vi "ModuleAction.Utility.vi"() -> ()   [LabVIEW 2014]
uses:
  <userlib>/_OpenG.lib/file/file.llb/Strip Path - Traditional__ogtk.vi
panel:
  in  "Stop Button":bool
  in  "Disk Properties":T1
  in  "Action Descriptor":T2
  out "Preview":string
  in  "Write to Disk":bool
  in  "Refresh":bool caption="Blank Button"
  out "Constructed Module Action Descriptor Location:":string
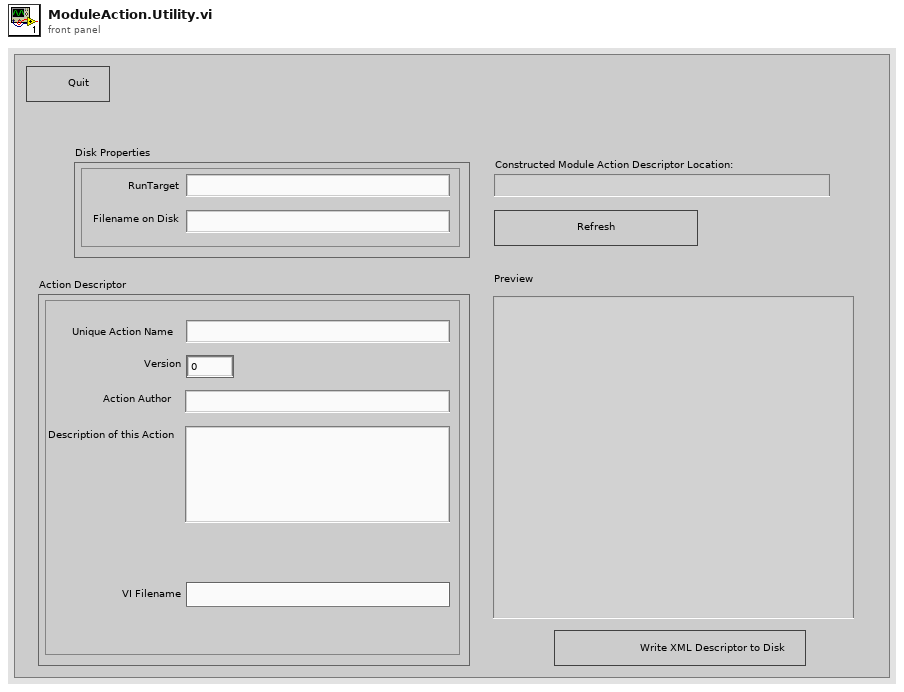
[diagram p1: front panel]
types:
  T1 = cluster{"RunTarget":string, "Filename on Disk":string}
  T2 = cluster{"Unique Action Name":string, "Version":dbl, "VI Filename":string, "Action Author":string, "Description of this Action":string}
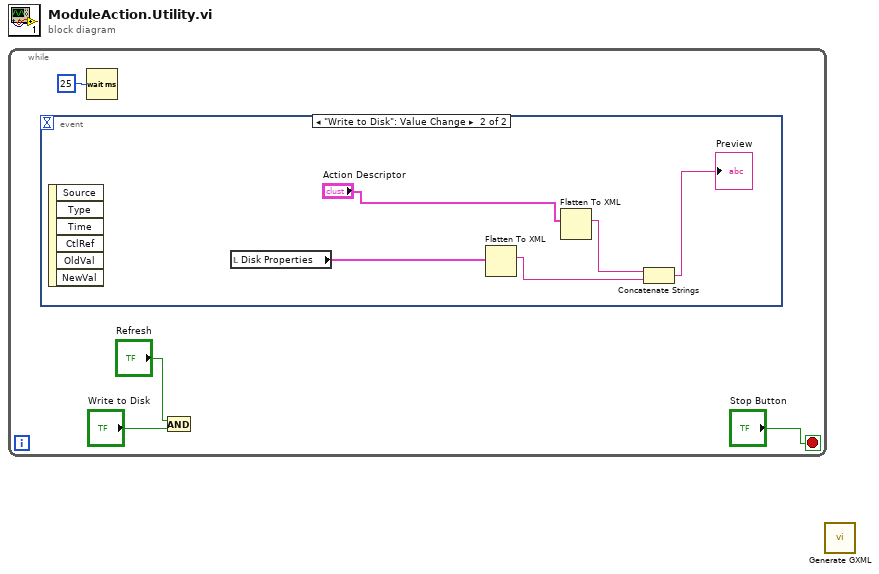
[diagram p0: block diagram]
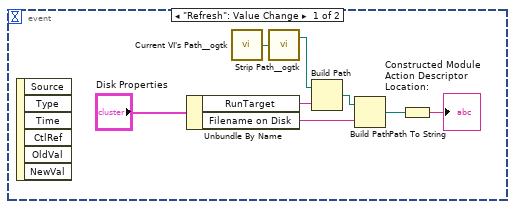
[diagram p2: hidden frame]
diagram:
  n1 = while {
    stop <- "Stop Button" stop-if-true
    n2 = event shown="[1] \"Write to Disk\": Value Change" {
      selector: _ -> [_ _]
      dyn-events: _ -> [_ _]
      timeout: _ -> [_ _]
      event "Refresh": Value Change {
        n3 = event-data() -> ()  [unwired: 1 in, 6 out]
        n4 = Unbundle By Name("Disk Properties") -> ("RunTarget"=w9:string, "Filename on Disk"=w7:string)
        n5 = call <userlib>:"Current VI's Path__ogtk.vi"() -> ("Current VI's Path (+ Relative)"=w11:path)  [unwired: 1 in]
        n6 = call-poly <userlib>:"Strip Path__ogtk.vi"("path"=w11) -> ("stripped path"=w10:path)  [unwired: 1 out]
        n7 = Build Path(base path=w10, name or relative path=w9) -> (appended path=w8:path)
        n8 = Build Path(base path=w8, name or relative path=w7) -> (appended path=w6:path)
        n9 = Path To String(path=w6) -> (string=→"Constructed Module Action Descriptor Location:":string)
      }
      event "Write to Disk": Value Change {
        n10 = event-data() -> ()  [unwired: 1 in, 6 out]
        n11 = local read "Disk Properties"() -> (w14:T1)
        n12 = Flatten To XML(anything=w14) -> (xml string=w13:string)
        n13 = Flatten To XML(anything="Action Descriptor") -> (xml string=w15:string)
        n14 = Concatenate Strings(w15, w13) -> (→"Preview":string)
      }
    }
    n15 = Wait (ms)(milliseconds to wait=u32 25) -> ()  [unwired: 1 out]
    n16 = And(x="Refresh", y="Write to Disk") -> ()  [unwired: 1 out]
  }
  n17 = call <vilib>:"Generate GXML.vi"() -> ()  [unwired: 1 in]
